vi "Initialize.vi"(8 "error in":errorcluster, 10 "port":u16, 11 "server in":refnum<class "RT FlexRIO Server TCP.lvclass">) -> (0 "error out":errorcluster, 3 "server in":refnum<class "RT FlexRIO Server TCP.lvclass">)   [LabVIEW 2017, in "RT FlexRIO Server TCP.lvclass"]
uses:
  RT FlexRIO Server TCP.lvclass
  Private/SessionData.ctl
  State.ctl
  RT FlexRIO Server TCP.lvclass/RT FlexRIO Server TCP.ctl
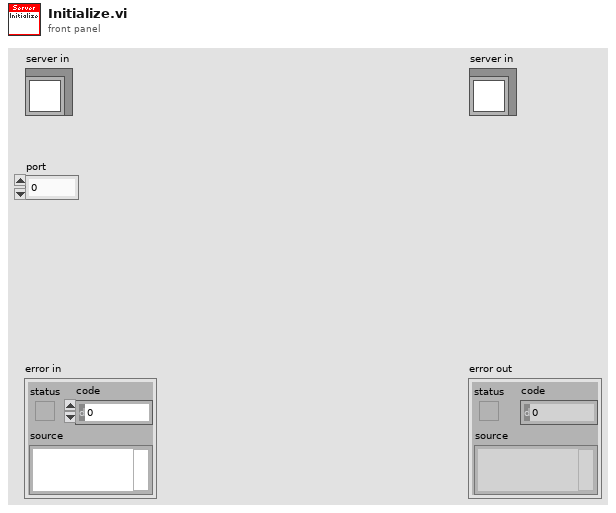
[diagram p1: front panel]
types:
  T1 = typedef "RT FlexRIO Server TCP.lvclass/State.ctl" = enum16{"started", "connected", "stopped"}
  T2 = typedef "RT FlexRIO Server TCP.lvclass/SessionData.ctl" = cluster{"listener":refnum<k5>, "connection":refnum<k5>, "state":T1, "incoming":refnum<queue>, "outgoing":refnum<queue>, "state request":refnum<user-event>, "state changed":refnum<user-event>}
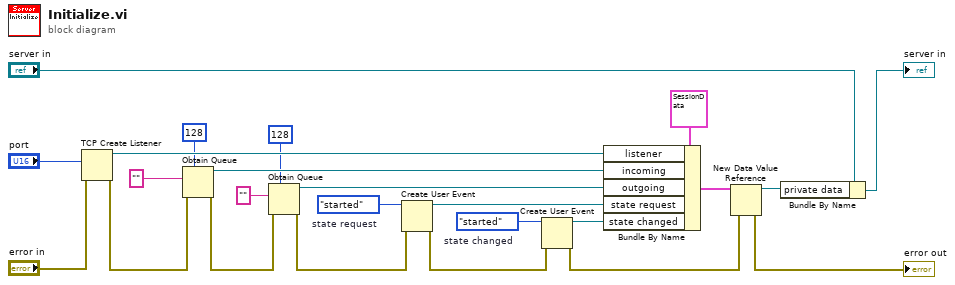
[diagram p0: block diagram]
diagram:
  w5 = State."started"  # state request
  w8 = State."started"  # state changed
  n1 = TCP Create Listener(8:"error in", 10:"port") -> (0:w17:errorcluster, 3:w20:refnum<k5>)  [unwired: 3 in, 1 out]
  n2 = Obtain Queue(max queue size (-1, unlimited)=128, element data type="", error in (no error)=w17) -> (queue out=w15:refnum<queue>, error out=w14:errorcluster)  [unwired: 2 in, 1 out]
  n3 = Obtain Queue(max queue size (-1, unlimited)=128, element data type="", error in (no error)=w14) -> (queue out=w13:refnum<queue>, error out=w11:errorcluster)  [unwired: 2 in, 1 out]
  n4 = Create User Event(user event datatype=w5, error in=w11) -> (user event=w6:refnum<user-event>, error out=w10:errorcluster)
  n5 = Create User Event(user event datatype=w8, error in=w10) -> (user event=w7:refnum<user-event>, error out=w9:errorcluster)
  n6 = Bundle By Name(cluster=T2 {"listener"=refnum, "connection"=refnum, "state"=enum."started", "incoming"=refnum, "outgoing"=refnum, "state request"=refnum, "state changed"=refnum} ("sessionData"), "listener"=w20, "incoming"=w15, "outgoing"=w13, "state request"=w6, "state changed"=w7) -> (w21:T2)
  n7 = New Data Value Reference(data value=w21, error in=w9) -> (data value reference=w18:refnum<data-value>, error out=→"error out":errorcluster)
  n8 = Bundle By Name(cluster="server in", "private data"=w18) -> (→"server in":refnum<class "RT FlexRIO Server TCP.lvclass">)
